vi "LinearSystemSim_UpdateX.vi"(6 "dT_Seconds":dbl=0.02, 9 "U":T1, 10 "CurrentXHat":T1, 11 "in LinearSystem":T2) -> (0 "Error":bool, 3 "X":T1)   [LabVIEW 2019, in "Trajectory_Library.lvlib"]
doc: "Updates the state estimate of the system.\n \nInputs:\n - LinearSystem -- Data cluster\n - currentXhat -- The current state estimate.\n - u -- The system inputs (usually voltage).\n - dtSeconds -- The time difference between controller updates.\n\nOutputs:\n - X -- The new state.\n - Error -- If TRUE, an error occured."
uses:
  Trajectory_Library.lvlib
  TypeDef/LINEAR_SYSTEM.ctl
  <vilib>/Analysis/Matrix/Datatypes/RealMatrix.ctl
  Discretization_DiscretizeAB.vi
  <vilib>/Analysis/baseanly.llb/A x B.vi
  <vilib>/Analysis/baseanly.llb/Real A x B.vi
  MatrixHelper_CoerceSize.vi
  MatBuilder_Create.vi
  Matrix_Exp.vi
  Matrix_AssignBlock.vi
  Matrix_ExtractFrom.vi
  <vilib>/Analysis/7linalg.llb/Matrix Exp.vi
  <vilib>/Analysis/7linalg.llb/Real Matrix Exp.vi
  <vilib>/Analysis/Matrix/Numeric/Multiply/Multiply.vi
  <vilib>/Analysis/Matrix/Numeric/Multiply/Multiply - RM,R.vi
  <vilib>/Analysis/Matrix/Numeric/Add/Add.vi
  <vilib>/Analysis/Matrix/Numeric/Add/Add - RM,RM.vi
  <vilib>/Analysis/Matrix/NI_Matrix.lvlib
panel:
  # "<States,States>"
  # "<States,Inputs>"
  # "<Outputs,States>"
  # "<Outputs,Inputs>"
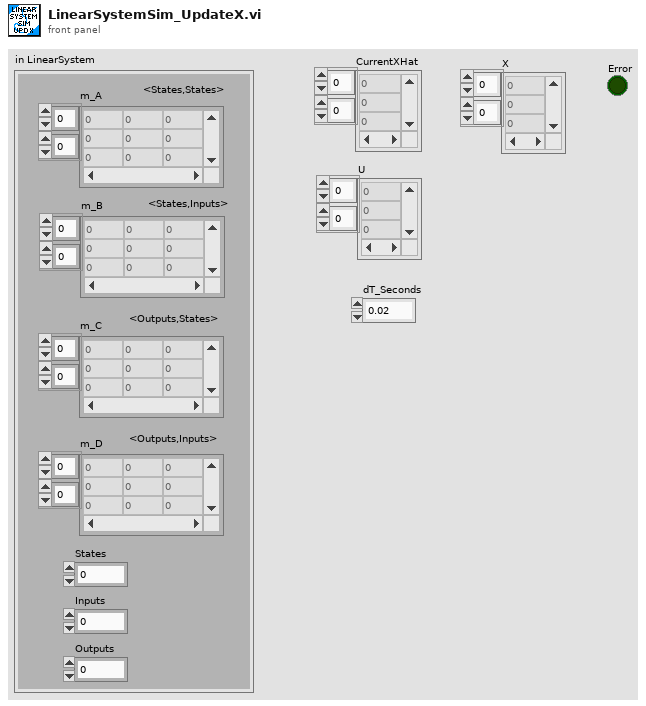
[diagram p1: front panel]
types:
  T1 = typedef "NI_Matrix.lvlib/RealMatrix.ctl" = dbl[][]
  T2 = typedef "Trajectory_Library.lvlib/LINEAR_SYSTEM.ctl" = cluster{"m_A":T1, "m_B":T1, "m_C":T1, "m_D":T1, "States":i32, "Inputs":i32, "Outputs":i32}
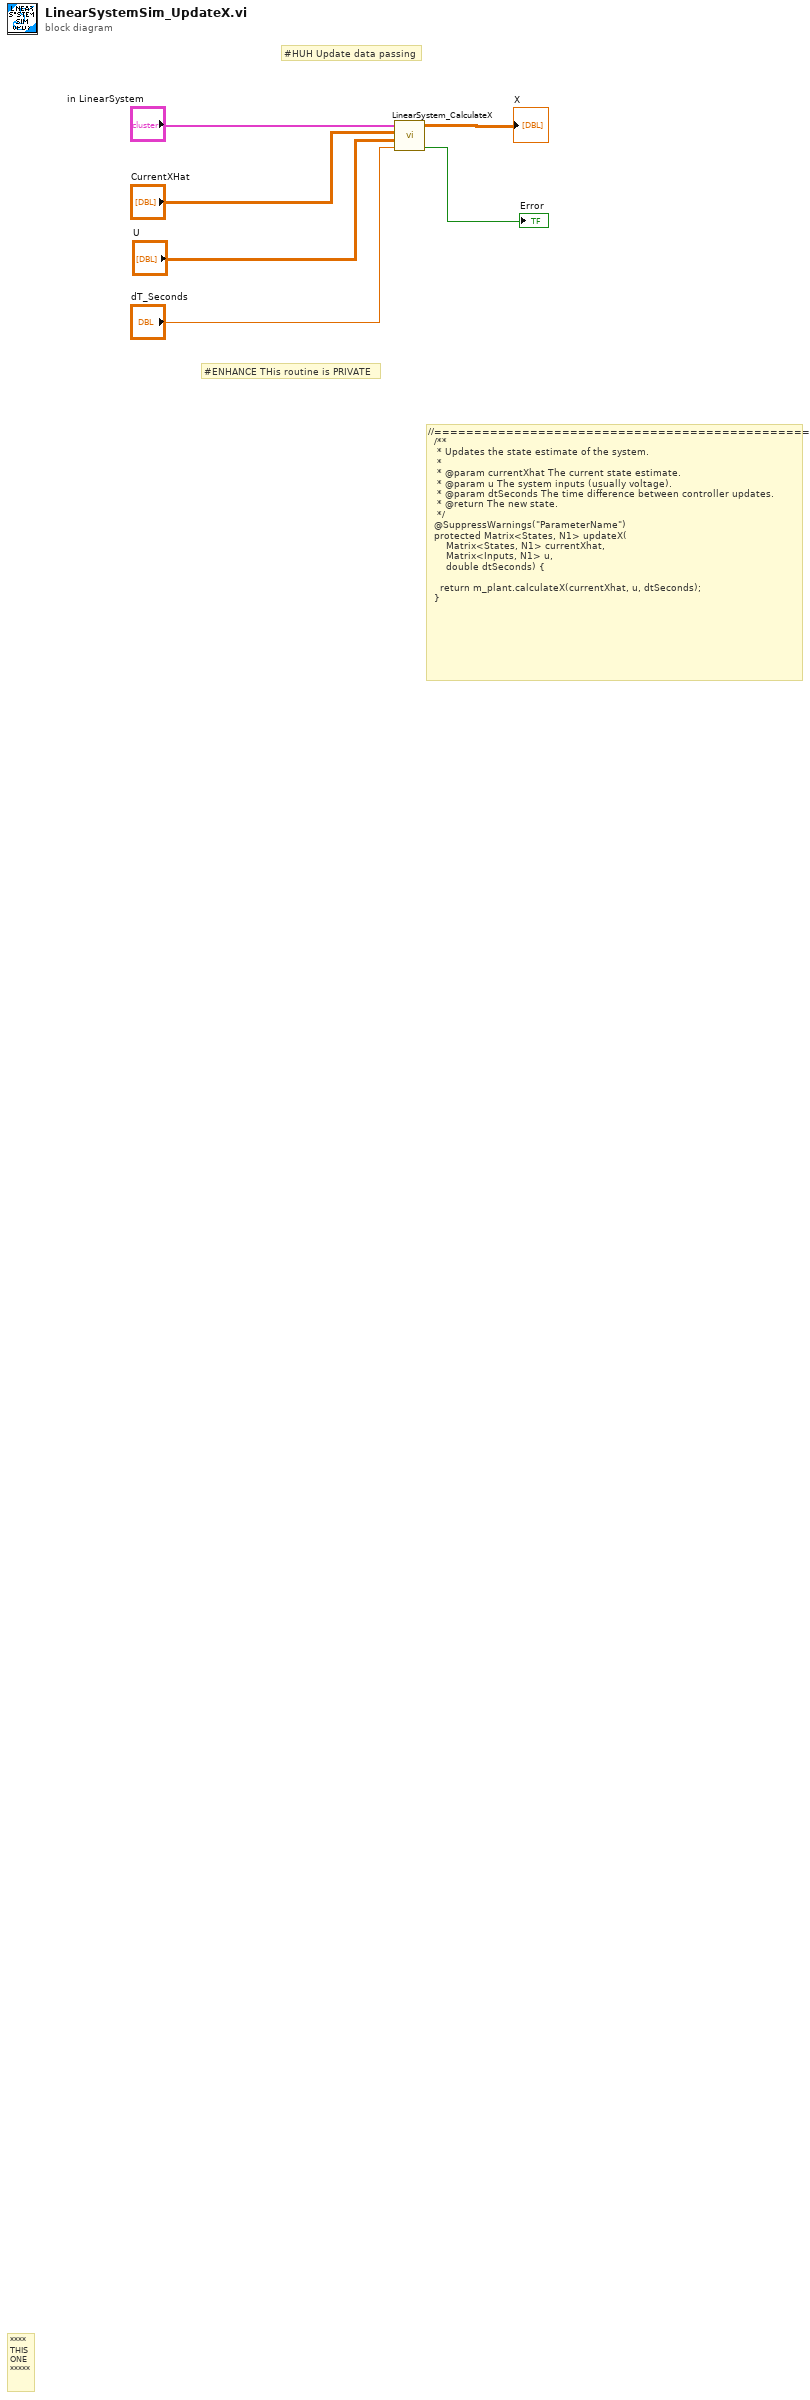
[diagram p0: block diagram]
diagram:
  # "#HUH Update data passing"
  # "#ENHANCE THis routine is PRIVATE"
  # "//================================================\n  /**\n   * Updates the state estimate of the system.\n   *\n   * @param currentXhat The current state estimate.\n   * @param u The system inputs (usually voltage).\n   * @param dtSeconds The time difference between controller updates.\n   * @return The new state.\n   */\n  @SuppressWarnings(\"ParameterName\")\n  protected Matrix<States, N1> updateX(\n      Matrix<States, N1> currentXhat, \n      Matrix<Inputs, N1> u, \n      double dtSeconds) {\n\n    return m_plant.calculateX(currentXhat, u, dtSeconds);\n  }"
  # "****\nTHIS\nONE\n*****"
  n1 = call "LinearSystem_CalculateX.vi"("dT_Seconds"="dT_Seconds", "ClampedU"="U", "X"="CurrentXHat", "Linearsystem"="in LinearSystem") -> ("Error"=→"Error":bool, "outX"=→"X":T1)  [unwired: 6 in]
